vi "calibration_image_to_conversion_ratio.vi"(8 "error in (no error)":errorcluster, 10 "Calibration Image":T1) -> (0 "error out":errorcluster, 2 "conversion ratio":dbl)   [LabVIEW 2019]
uses:
  <vilib>/vision/Image Controls.llb/IMAQ Image.ctl
  <vilib>/vision/NI_Vision_Development_Module.lvlib
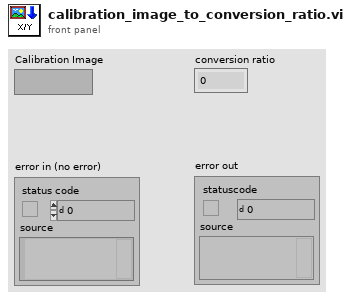
[diagram p1: front panel]
types:
  T1 = typedef "IMAQ Image.ctl" = refnum<image>
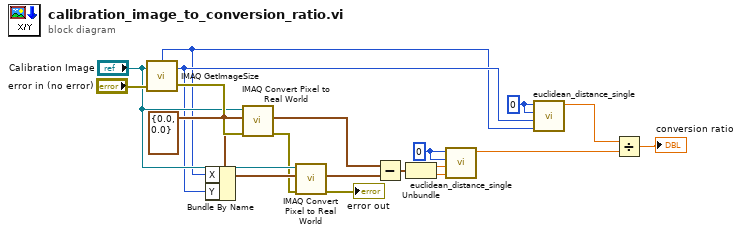
[diagram p0: block diagram]
diagram:
  w12 = 0
  w13 = 0
  w17 = cluster{"X":dbl, "Y":dbl} {"X"=0.0, "Y"=0.0}
  n1 = call "IMAQ GetImageSize"("Image"="Calibration Image", "error in (no error)"="error in (no error)") -> ("Y Resolution"=w6:i32, "X Resolution"=w5:i32, "error out"=w18:errorcluster)  [unwired: 2 in]
  n2 = Bundle By Name(cluster=w17, "X"=w5, "Y"=w6) -> (w15:cluster{"X":dbl, "Y":dbl})
  n3 = call "IMAQ Convert Pixel to Real World"("error in (no error)"=w18, "Pixel Coordinates"=w17, "Calibrated Image"="Calibration Image") -> ("error out"=w14:errorcluster, "Real World Coordinates"=w11:cluster{"X":sgl, "Y":sgl})  [unwired: 3 in, 4 out]
  n4 = call "IMAQ Convert Pixel to Real World"("error in (no error)"=w14, "Pixel Coordinates"=w15, "Calibrated Image"="Calibration Image") -> ("error out"=→"error out":errorcluster, "Real World Coordinates"=w10:cluster{"X":sgl, "Y":sgl})  [unwired: 3 in, 4 out]
  n5 = Subtract(x=w11, y=w10) -> (x-y=w9:cluster{"X":sgl, "Y":sgl})
  n6 = Unbundle(w9) -> ("X"=w8:sgl, "Y"=w7:sgl)
  n7 = call "euclidean_distance_single.vi"("Point 2 Y"=w7, "Point 2 X"=w8, "Point 1 Y"=w12, "Point 1 X"=w12) -> ("Distance"=w2:sgl)  [unwired: 7 in]
  n8 = call "euclidean_distance_single.vi"("Point 2 Y"=w5, "Point 2 X"=w6, "Point 1 Y"=w13, "Point 1 X"=w13) -> ("Distance"=w1:sgl)  [unwired: 7 in]
  n9 = Divide(x=w1, y=w2) -> (x/y=→"conversion ratio":sgl)
